vi "ssh_PuTTY.vi"(5 "Host":string="10.8.2.12", 7 "Username":string="tvt", 10 "plink.exe  path":path=path "C:/Program Files/PuTTY/plink.exe", 11 "Command(s) to Execute":string(combo)="pwd") -> (0 "Errors":string, 3 "Command Return Value(s)":string="/home/tvt\n")   [LabVIEW 2022 SP3]
panel:
  out "Command Executed":string="C:\\Program Files\\PuTTY\\plink.exe tvt@10.8.2.12 -ssh -pw TDDPc5kc4WnYcy -m D:\\scriptfile.txt"
  in  "Protocol":u16(ring)=2 items=["Telnet", "Rlogin", "SSH", "RAW"]
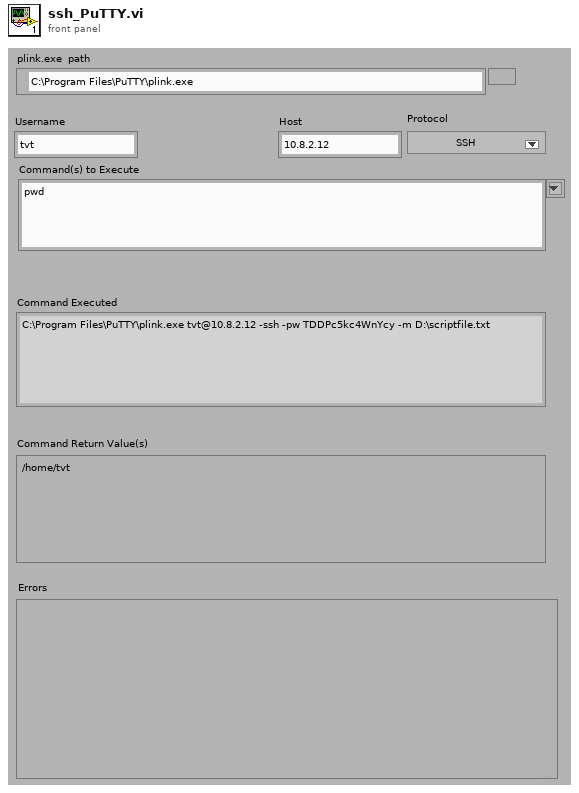
[diagram p1: front panel]
types:
  T1 = enum16{"open", "replace", "create", "open or create", "replace or create", "replace or create with confirmation"}
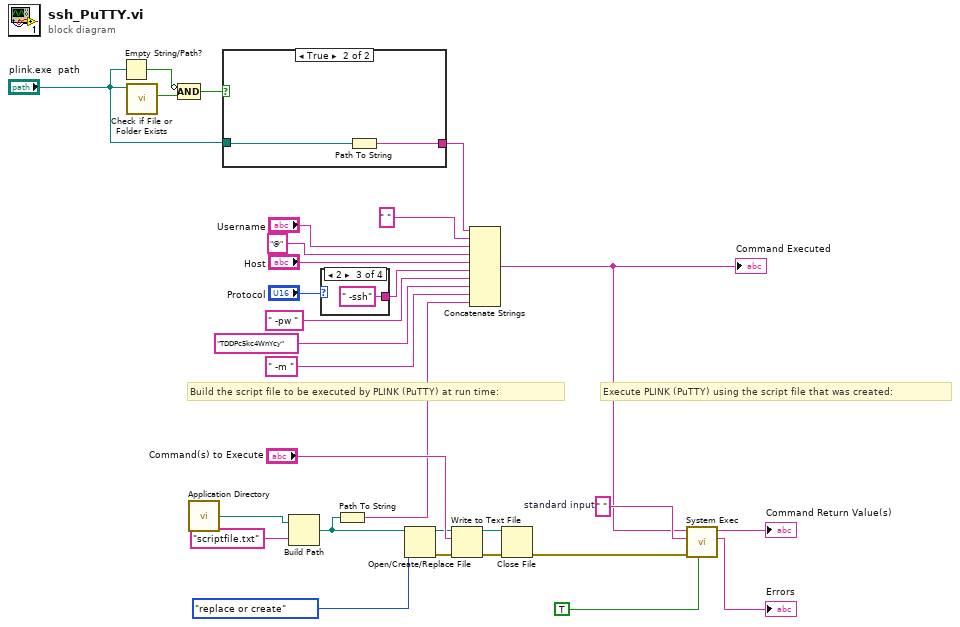
[diagram p0: block diagram]
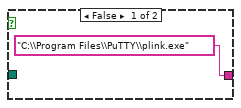
[diagram p2: hidden frame]
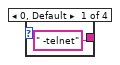
[diagram p3: hidden frame]
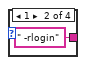
[diagram p4: hidden frame]
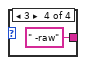
[diagram p5: hidden frame]
diagram:
  w22 = " "  # standard input
  # "Execute PLINK (PuTTY) using the script file that was created:"
  # "Build the script file to be executed by PLINK (PuTTY) at run time:"
  n1 = Empty String/Path?(string/path="plink.exe  path") -> (empty?=w1:bool)
  n2 = call <vilib>:"Check if File or Folder Exists.vi"("path"="plink.exe  path") -> ("file or folder exists?"=w5:bool)  [unwired: 8 in, 2 out]
  n3 = Compound Arithmetic op=AND(invert w1, w5) -> (w2:bool)
  n4 = call <vilib>:"Application Directory.vi"() -> ("Application Directory"=w6:path)
  n5 = case shown="True" w2 {
    tunnel: "plink.exe  path" -> [_ w33]
    tunnel: ["C:\\Program Files\\PuTTY\\plink.exe" w32] -> w4
    frame False {
    }
    frame True {
      n6 = Path To String(path=w33) -> (string=w32:string)
    }
  }
  n7 = Build Path(base path=w6, name or relative path="scriptfile.txt" ("command line")) -> (appended path=w8:path)
  n8 = case shown="2" "Protocol" {
    tunnel: [" -telnet" " -rlogin" " -ssh" " -raw"] -> w17
    frame 0, Default {
    }
    frame 1 {
    }
    frame 2 {
    }
    frame 3 {
    }
  }
  n9 = Path To String(path=w8) -> (string=w9:string)
  n10 = Open/Create/Replace File(file path (use dialog)=w8, operation (0:open)=T1."replace or create") -> (refnum out=w25:refnum<file>, error out=w24:errorcluster)  [unwired: 4 in, 1 out]
  n11 = Write to Text File(file (use dialog)=w25, text="Command(s) to Execute", error in=w24) -> (refnum out=w28:refnum<file>, error out=w27:errorcluster)  [unwired: 2 out]
  n12 = Concatenate Strings(w4, " ", "Username", "@" ("string"), "Host", w17, " -pw " ("string"), "TDDPc5kc4WnYcy" ("Password"), " -m " ("string"), w9) -> (w13:string)
  "Command Executed" <- w13
  n13 = Close File(refnum=w28, error in=w27) -> (error out=w26:errorcluster)  [unwired: 1 out]
  n14 = call <vilib>:"System Exec.vi"("run minimized? (F)"=TRUE ("Hide DOS\nWindow?"), "error in (no error)"=w26, "standard input"=w22, "command line"=w13) -> ("standard error"=→"Errors":string, "standard output"=→"Command Return Value(s)":string)  [unwired: 2 in, 4 out]
